vi "Check if at destination.vi"(8 "error in (no error)":errorcluster, 11 "StageSPIM in":refnum<class "StageSPIM.lvclass">) -> (0 "error out":errorcluster, 2 "at destination?":bool, 3 "StageSPIM out":refnum<class "StageSPIM.lvclass">)   [LabVIEW 2012, in "StageSPIM.lvclass"]
uses:
  StageSPIM.lvclass
  StageSPIM.lvclass/StageSPIM.ctl
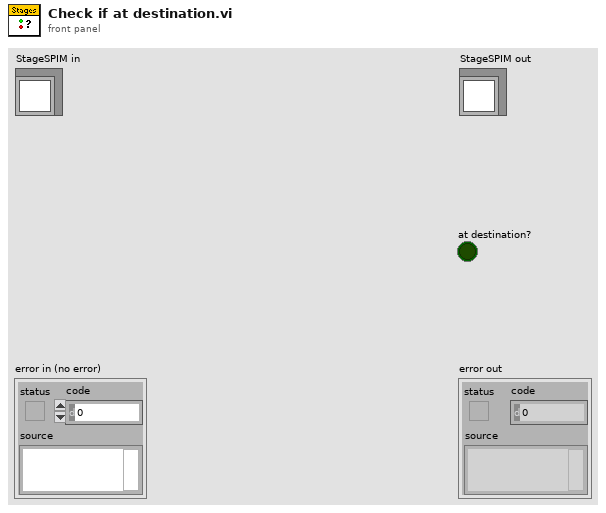
[diagram p1: front panel]
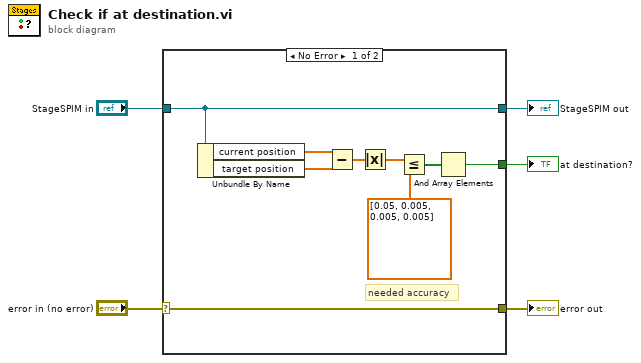
[diagram p0: block diagram]
diagram:
  n1 = case shown="No Error" "error in (no error)" {
    selector: "error in (no error)" -> [w14 w16]
    tunnel: [w14 w16] -> w4
    tunnel: [w13 w15] -> w2
    tunnel: "StageSPIM in" -> [w13 w15]
    tunnel: [w6 _] -> w1
    frame No Error {
      # "needed accuracy"
      n2 = Unbundle By Name(w13) -> ("current position"=w12:dbl[], "target position"=w11:dbl[])
      n3 = Subtract(x=w12, y=w11) -> (x-y=w10:dbl[])
      n4 = Absolute Value(x=w10) -> (abs(x)=w9:dbl[])
      n5 = Less Or Equal?(x=w9, y=dbl[] [0.05, 0.005, 0.005, 0.005]) -> (x <= y?=w7:bool[])
      n6 = And Array Elements(Boolean array=w7) -> (logical AND=w6:bool)
    }
    frame Error {
    }
  }
  "error out" <- w4
  "StageSPIM out" <- w2
  "at destination?" <- w1
